vi "RSZVB Start Noise Figure Calibration.vi"(8 "error in (no error)":errorcluster {"code" format="%.0x"}, 9 "Calibration Step (0)":i32(ring) items=["Receiver", "Source", "Attenuator"], 10 "Channel (1)":i32=1, 11 "VISA session":refnum<visa-resource-name>) -> (0 "error out":errorcluster {"code" format="%.0x"}, 3 "dup VISA session":refnum<visa-resource-name>)   [LabVIEW 2011]
doc: "This VI starts a noise figure calibration sweep for the NWA receiver, NWA source, or an external attenuator.\n\nNote(s):\n\n(1) This VI is available only with option R&S ZVAB-K30.\n\n(2) A noise figure calibration must be terminated with one of the following VIs, to be sent immediately after the sequence of ...[:ACQuire] commands: \n\nrszvb_TerminateNoiseFigureCalibration - terminate calibration, discarding the acquired calibration data (the active channel is not calibrated) \n\nrszvb_CompleteNoiseFigureCalibration - terminate calibration, applying the acquired calibration data (the active channel is calibrated) \n\nThese VIs ensure that the analyzer is able to start a new measurement sweep.\n\nRemote-control command(s):\n[SENSe<Ch>:]CORRection:COLLect:NFIGure[:ACQuire] RECeiver | SOURce | ATTenuator"
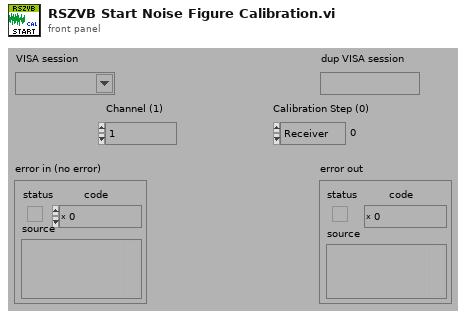
[diagram p1: front panel]
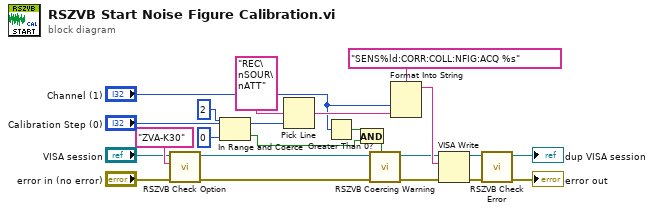
[diagram p0: block diagram]
diagram:
  n1 = call "RSZVB Check Option.vi"("error in (no error)"="error in (no error)", "Options"="ZVA-K30", "VISA session"="VISA session") -> ("error out"=w15:errorcluster, "dup VISA session"=w16:refnum<visa-resource-name>)  [unwired: 7 in]
  n2 = In Range and Coerce(upper limit=2, x="Calibration Step (0)", lower limit=0) -> (coerced(x)=w7:i32, In Range?=w1:bool)
  n3 = Pick Line(multi-line string="REC\nSOUR\nATT" ("string (\"\")"), line index=w7) -> (output string=w9:string)  [unwired: 1 in]
  n4 = Greater Than 0?(x="Channel (1)") -> (x > 0?=w3:bool)
  n5 = And(x=w3, y=w1) -> (x .and. y?=w2:bool)
  n6 = call "RSZVB Coercing Warning.vi"("In Range?"=w2, "error in (no error)"=w15, "VISA session"=w16) -> ("error out"=w21:errorcluster, "dup VISA session"=w20:refnum<visa-resource-name>)  [unwired: 7 in]
  n7 = Format Into String(format string="SENS%ld:CORR:COLL:NFIG:ACQ %s", "Channel (1)", w9) -> (resulting string=w22:string)  [unwired: 2 in, 1 out]
  n8 = VISA Write(VISA resource name=w20, write buffer=w22, error in (no error)=w21) -> (VISA resource name out=w17:refnum<visa-resource-name>, error out=w18:errorcluster)  [unwired: 1 out]
  n9 = call "RSZVB Check Error.vi"("error in (no error)"=w18, "VISA session"=w17) -> ("error out"=→"error out":errorcluster, "dup VISA session"=→"dup VISA session":refnum<visa-resource-name>)  [unwired: 8 in]
